vi "control - IMscram - increment buttons.vi"() -> ()   [LabVIEW 2017]
uses:
  <vilib>/imath/engines/lvmath2/RunTimeEngine/Managers/WorkSpace/UID Generator.vi
  Documents/LabVIEW Data/MathScriptVIs/MCStatic_38597427832_24a4e2d6858359c1fa390f3b06d361fe.vi
  <instcachedir>/0/MCStatic_38597427832_24a4e2d6858359c1fa390f3b06d361fe_53CC8FBD344742A8B22F0400F764026F.lvgen/MCStatic_38597427832_24a4e2d6858359c1fa390f3b06d361fe_53CC8FBD344742A8B22F0400F764026F_000.vi
  <vilib>/imath/engines/lvmath2/RunTimeEngine/RunTimeType/NIMS_RunTimeType_From StrictType (excl LVString).vi
  <instcachedir>/0/NIMS_RunTimeType_From StrictType (excl LVString)_1019F277F0A747EDBCA0F6C52CA54500.lvgen/NIMS_RunTimeType_From StrictType (excl LVString)_1019F277F0A747EDBCA0F6C52CA54500_000.vi
  <vilib>/imath/engines/lvmath2/RunTimeEngine/RunTimeType/NIMS_RunTimeType_Set Source Original Bool.vi
  <vilib>/imath/engines/lvmath2/RunTimeEngine/LocalVariableDefStatement/MC_LocalVariableDefStatement_Display.vi
  <vilib>/imath/engines/lvmath2/RunTimeEngine/Managers/SymbolTable/Clear UID.vi
  <vilib>/imath/engines/lvmath2/RunTimeEngine/NodeEndStatement/NIMS_NodeEndStatement_Output.vi
  <instcachedir>/0/NIMS_NodeEndStatement_Output_53EC0D466D134D7ABD903AC30B43404B.lvgen/NIMS_NodeEndStatement_Output_53EC0D466D134D7ABD903AC30B43404B_001.vi
  <instcachedir>/0/NIMS_NodeEndStatement_Output_53EC0D466D134D7ABD903AC30B43404B.lvgen/NIMS_NodeEndStatement_Output_53EC0D466D134D7ABD903AC30B43404B_010.vi
  <instcachedir>/0/NIMS_NodeEndStatement_Output_53EC0D466D134D7ABD903AC30B43404B.lvgen/NIMS_NodeEndStatement_Output_53EC0D466D134D7ABD903AC30B43404B_002.vi
  <vilib>/imath/engines/lvmath2/RunTimeEngine/ErrorHandling/NIMS_Finalize Error.vi
  Documents/LabVIEW Data/MathScriptVIs/MCStatic_38597427832_80100019c1ecfa069c897e41bc996adc.vi
  <instcachedir>/0/MCStatic_38597427832_80100019c1ecfa069c897e41bc996adc_8B88C90F0EB544718CCB48C9924978D1.lvgen/MCStatic_38597427832_80100019c1ecfa069c897e41bc996adc_8B88C90F0EB544718CCB48C9924978D1_001.vi
  Documents/LabVIEW Data/read2.m
  Documents/LabVIEW Data/reactor_power.m
  Documents/LabVIEW Data/long_term_power.m
  Documents/LabVIEW Data/power_function.m
  <vilib>/imath/engines/lvmath2/RunTimeEngine/Managers/SymbolTable/NIMS_WorkSpace.lvlib
panel:
  in  "Select Operation Mode":i32
  in  "Power Output On":bool
  out "Power":dbl
  out "BT-11":sgl
  out "ST-13":sgl
  out "Max k Value":dbl
  out "k value":dbl
  out "Reactivity":dbl
  in  "Fine":bool
  out "Waveform Chart":dbl(graph)
  out "Increasing?":bool
  in  "Decrease":bool
  out "Decreasing?":bool
  in  "Increase":bool
  out "Time (s)":dbl caption="Elapsed Time (s)"
  out "Iteration":i32
  out "Controlled rods out":dbl
  out "Go Scram":bool
  out "Time Satisfied":bool
  out "on":bool
  out "reset":dbl
  in  "Scram":bool
  out "Delta Satisfied":bool
  out "IM delta":dbl
  out "IM Scram Mechanism":dbl[][](array[numeric])
  out "Control Rods Positioning":dbl[][](array[numeric])
  out "Rods out":dbl format="%#_9g"
  out "Max rods out":dbl format="%#_9g"
  in  "Stop":bool
  # "MAIN WINDOW"
  # "Actual Values"
  # "Maximum Values"
  # "0 = Resistance Feedback\n2 = Shutdown"
  # "Double tap & hold"
  # "Averages"
  # "Hard1"
  # "Med1"
  # "Soft1"
  # "Hard2"
  # "Med2"
  # "Soft2"
  # "Hard3"
  # "Med3"
  # "Soft3"
  # "Initiator"
  # "Mover"
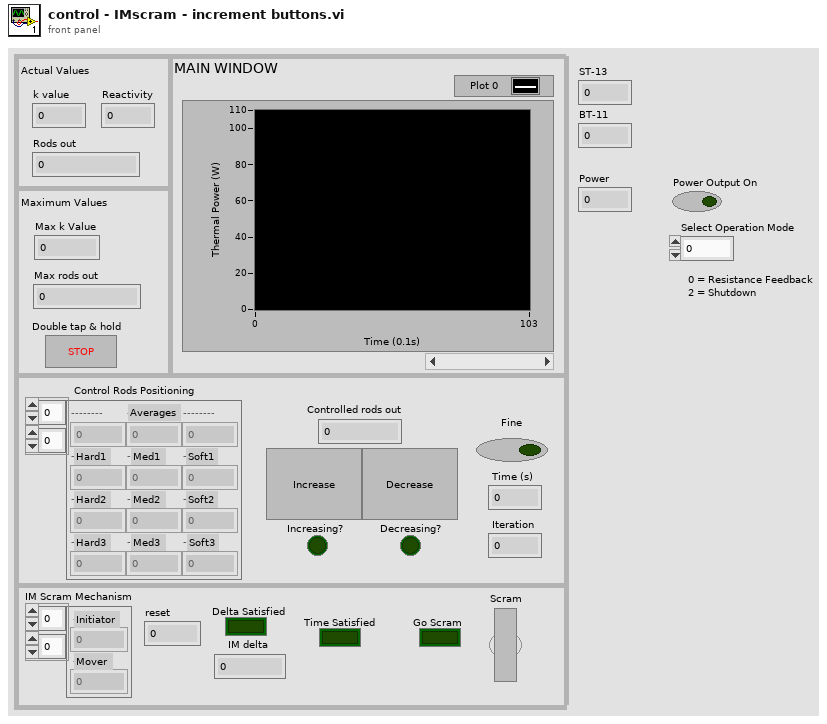
[diagram p1: front panel]
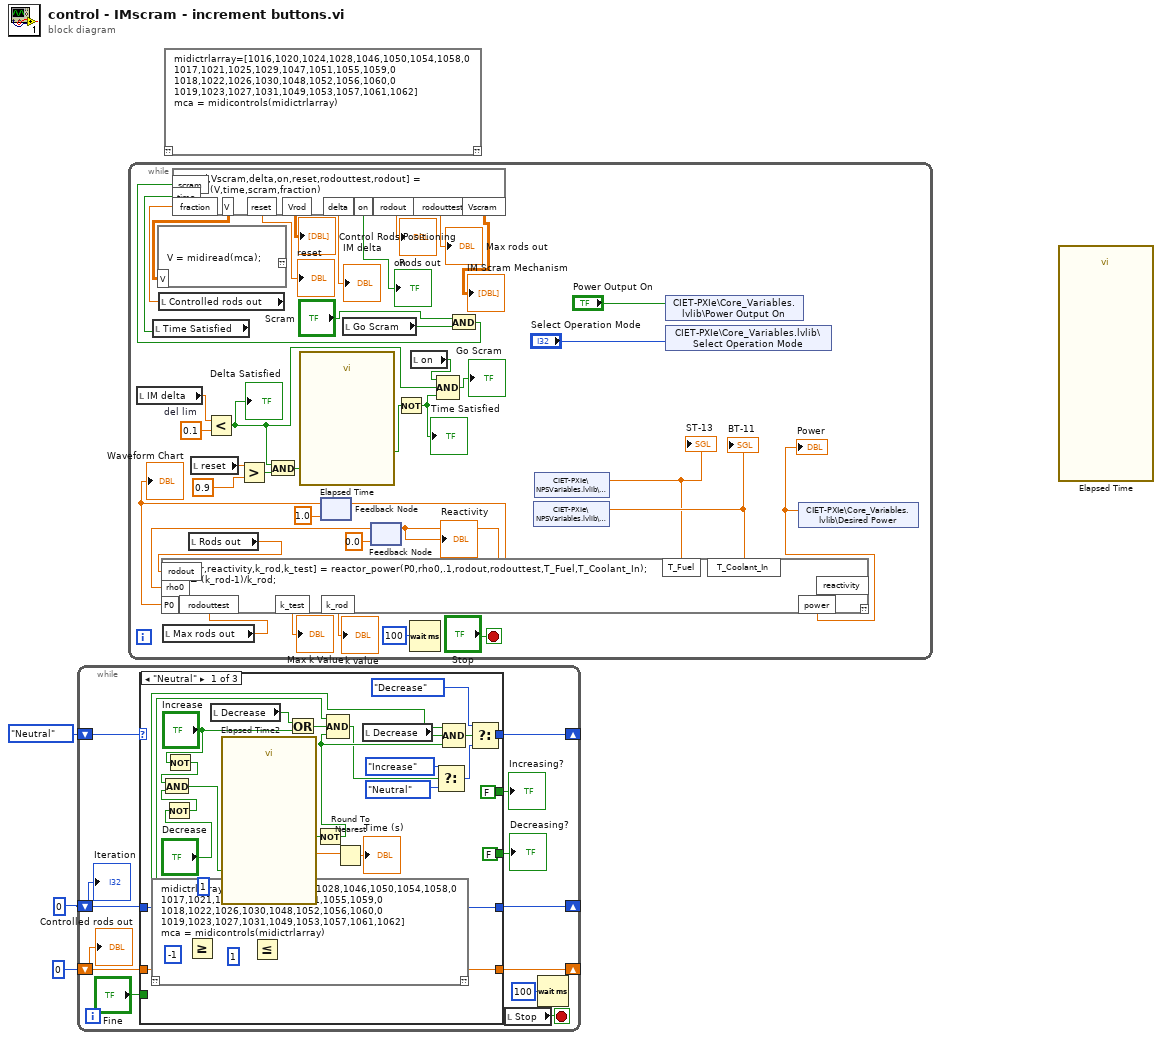
[diagram p0: block diagram]
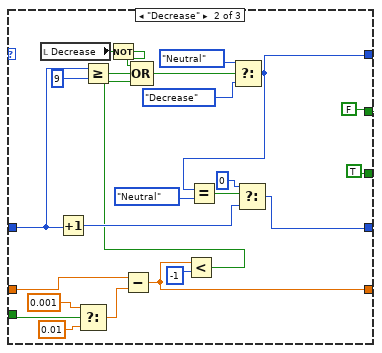
[diagram p2: hidden frame]
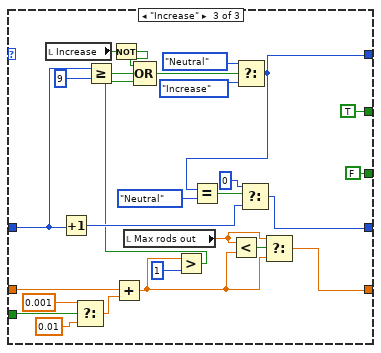
[diagram p3: hidden frame]
diagram:
  n1 = while {
    shift-right: [w12] -> _
    shift-left: enum16{"Increase", "Neutral", "Decrease"}."Neutral" -> [w13]
    shift-right: [w10] -> _
    shift-left: 0 -> [w11]
    shift-right: [w5] -> _
    shift-left: 0 -> [w8]
    stop <- w9 stop-if-true
    n2 = case shown="\"Neutral\"" w13 {
      tunnel: [w33 w49 w86] -> w12
      tunnel: w11 -> [w39 w51 w92]
      tunnel: [w39 w50 w84] -> w10
      tunnel: w8 -> [w15 w47 w69]
      tunnel: [w15 w48 w72] -> w5
      tunnel: [FALSE FALSE TRUE] -> w7
      tunnel: [FALSE TRUE FALSE] -> w6
      tunnel: "Fine" -> [_ w44 w68]
      frame "Neutral" {
        n3 = Not(x="Decrease") -> (.not. x?=w32:bool)
        n4 = Not(x="Increase") -> (.not. x?=w34:bool)
        n5 = And(x=w34, y=w32) -> (x .and. y?=w30:bool)
        n6 = Greater Or Equal?(x=w15, y=-1) -> (x >= y?=w17:bool)
        n7 = local read "Decrease"() -> (w24:bool)
        n8 = call "Elapsed Time2"("Time Target (s)"=1, "Reset"=w30) -> ("Elapsed Time (s)"=w38:dbl, "Time has Elapsed"=w40:bool)  [unwired: 10 in, 6 out]
        n9 = Less Or Equal?(x=w15, y=1) -> (x <= y?=w21:bool)
        n10 = Or(x=w24, y="Increase") -> (x .or. y?=w23:bool)
        n11 = Not(x=w40) -> (.not. x?=w20:bool)
        n12 = Compound Arithmetic op=AND(w21, w23, w20) -> (w18:bool)
        n13 = Round To Nearest(number=w38) -> (nearest integer value=→"Time (s)":dbl)
        n14 = local read "Decrease"() -> (w19:bool)
        n15 = Select(t=enum16{"Increase", "Neutral", "Decrease"}."Increase", s=w18, f=enum16{"Increase", "Neutral", "Decrease"}."Neutral") -> (s? t:f=w26:enum16{"Increase", "Neutral", "Decrease"})
        n16 = Compound Arithmetic op=AND(w17, w19, w20) -> (w22:bool)
        n17 = Select(t=enum16{"Increase", "Neutral", "Decrease"}."Decrease", s=w22, f=w26) -> (s? t:f=w33:enum16{"Increase", "Neutral", "Decrease"})
      }
      frame "Decrease" {
        n18 = local read "Decrease"() -> (w60:bool)
        n19 = Increment(x=w51) -> (x+1=w63:i32)
        n20 = Select(t=0.001, s=w44, f=0.01) -> (s? t:f=w43:dbl)
        n21 = Greater Or Equal?(x=w51, y=9) -> (x >= y?=w58:bool)
        n22 = Not(x=w60) -> (.not. x?=w59:bool)
        n23 = Subtract(x=w47, y=w43) -> (x-y=w48:dbl)
        n24 = Less?(x=w48, y=-1) -> (x < y?=w55:bool)
        n25 = Compound Arithmetic op=OR(w59, w58, w55) -> (w57:bool)
        n26 = Select(t=enum16{"Increase", "Neutral", "Decrease"}."Neutral", s=w57, f=enum16{"Increase", "Neutral", "Decrease"}."Decrease") -> (s? t:f=w49:enum16{"Increase", "Neutral", "Decrease"})
        n27 = Equal?(x=w49, y=enum16{"Increase", "Neutral", "Decrease"}."Neutral") -> (x = y?=w62:bool)
        n28 = Select(t=0, s=w62, f=w63) -> (s? t:f=w50:i32)
      }
      frame "Increase" {
        n29 = local read "Increase"() -> (w83:bool)
        n30 = Increment(x=w92) -> (x+1=w89:i32)
        n31 = Select(t=0.001, s=w68, f=0.01) -> (s? t:f=w67:dbl)
        n32 = Greater Or Equal?(x=w92, y=9) -> (x >= y?=w81:bool)
        n33 = Not(x=w83) -> (.not. x?=w82:bool)
        n34 = Add(x=w69, y=w67) -> (x+y=w73:dbl)
        n35 = local read "Max rods out"() -> (w74:dbl)
        n36 = Greater?(x=w73, y=1) -> (0:w78:bool)
        n37 = Compound Arithmetic op=OR(w82, w81, w78) -> (w80:bool)
        n38 = Less?(x=w74, y=w73) -> (x < y?=w75:bool)
        n39 = Select(t=enum16{"Increase", "Neutral", "Decrease"}."Neutral", s=w80, f=enum16{"Increase", "Neutral", "Decrease"}."Increase") -> (s? t:f=w86:enum16{"Increase", "Neutral", "Decrease"})
        n40 = Equal?(x=w86, y=enum16{"Increase", "Neutral", "Decrease"}."Neutral") -> (x = y?=w88:bool)
        n41 = Select(t=0, s=w88, f=w89) -> (s? t:f=w84:i32)
        n42 = Select(t=w74, s=w75, f=w73) -> (s? t:f=w72:dbl)
      }
    }
    "Increasing?" <- w7
    "Decreasing?" <- w6
    n43 = local read "Stop"() -> (w9:bool)
    n44 = Wait (ms)(milliseconds to wait=u32 100) -> ()  [unwired: 1 out]
    "Iteration" <- w11
    "Controlled rods out" <- w8
  }
  n45 = while {
    stop <- "Stop" stop-if-true
    w130 = 0.1  # del lim
    n46 = local read "IM delta"() -> (w131:dbl)
    n47 = local read "Time Satisfied"() -> (w116:bool)
    n48 = script code="V = midiread(mca);"() -> ("V"=w117:dbl[][])  [unwired: 1 in, 1 out]
    n49 = local read "Controlled rods out"() -> (w103:dbl)
    n50 = local read "Max rods out"() -> (w100:dbl)
    n51 = local read "Rods out"() -> (w104:dbl)
    n52 = local read "reset"() -> (w126:dbl)
    n53 = Less?(x=w131, y=w130) -> (x < y?=w110:bool)
    "Delta Satisfied" <- w110
    n54 = Greater?(x=w126, y=0.9) -> (0:w125:bool)
    n55 = And(x=w110, y=w125) -> (x .and. y?=w127:bool)
    n56 = call "Elapsed Time"("Reset"=w127) -> ("Time has Elapsed"=w128:bool)  [unwired: 11 in, 7 out]
    n57 = feedback #1(1.0 ("power")) -> (w105:dbl)
    "Waveform Chart" <- w105
    n58 = local read "Go Scram"() -> (w123:bool)
    n59 = feedback #2(0.0 ("reactivity")) -> (w108:dbl)
    n60 = Not(x=w128) -> (.not. x?=w115:bool)
    "Time Satisfied" <- w115
    n61 = Wait (ms)(milliseconds to wait=100) -> ()  [unwired: 1 out]
    n62 = local read "on"() -> (w112:bool)
    n63 = Compound Arithmetic op=AND(w112, w110, w115) -> (→"Go Scram":bool)
    n64 = And(x="Scram", y=w123) -> (x .and. y?=w109:bool)
    n65 = mathscript code="[Vrod,Vscram,delta,on,reset,rodouttest,rodout] = read2(V,time,scram,fraction)"("V"=w117, "scram"=w109, "time"=w116, "fraction"=w103) -> ("rodout"=→"Rods out":dbl, "rodouttest"=→"Max rods out":dbl, "Vrod"=→"Control Rods Positioning":dbl[][], "Vscram"=→"IM Scram Mechanism":dbl[][], "delta"=→"IM delta":dbl, "on"=→"on":bool, "reset"=→"reset":dbl)  [unwired: 1 in, 1 out]
    n66 = shared-variable "CIET-PXIe\\NPSVariables.lvlib\\BT-11"() -> (w98:sgl)  [unwired: 1 in, 1 out]
    "BT-11" <- w98
    n67 = shared-variable "CIET-PXIe\\NPSVariables.lvlib\\ST-13"() -> (w97:sgl)  [unwired: 1 in, 1 out]
    "ST-13" <- w97
    n68 = mathscript code="[power,reactivity,k_rod,k_test] = reactor_power(P0,rho0,.1,rodout,rodouttest,T_Fuel,T_Coolant_In);\nrho = (k_rod-1)/k_rod;"("P0"=w105, "rho0"=w108, "rodout"=w104, "rodouttest"=w100, "T_Fuel"=w97, "T_Coolant_In"=w98) -> ("power"=w96:dbl, "reactivity"=w102:dbl, "k_rod"=→"k value":dbl, "k_test"=→"Max k Value":dbl)  [unwired: 1 in, 1 out]
    "Reactivity" <- w102
    "Power" <- w96
    n69 = feedback-in #1(w96) -> ()
    n70 = feedback-in #2(w102) -> ()
    n71 = shared-variable "CIET-PXIe\\Core_Variables.lvlib\\Power Output On"("Power Output On") -> ()  [unwired: 1 in, 1 out]
    n72 = shared-variable "CIET-PXIe\\Core_Variables.lvlib\\Select Operation Mode"("Select Operation Mode") -> ()  [unwired: 1 in, 1 out]
    n73 = shared-variable "CIET-PXIe\\Core_Variables.lvlib\\Desired Power"(w96) -> ()  [unwired: 1 in, 1 out]
  }
  n74 = script code="midictrlarray=[1016,1020,1024,1028,1046,1050,1054,1058,0\n1017,1021,1025,1029,1047,1051,1055,1059,0\n1018,1022,1026,1030,1048,1052,1056,1060,0\n1019,1023,1027,1031,1049,1053,1057,1061,1062]\nmca = midicontrols(midictrlarray)"() -> ()  [unwired: 1 in, 1 out]
  n75 = script code="midictrlarray=[1016,1020,1024,1028,1046,1050,1054,1058,0\n1017,1021,1025,1029,1047,1051,1055,1059,0\n1018,1022,1026,1030,1048,1052,1056,1060,0\n1019,1023,1027,1031,1049,1053,1057,1061,1062]\nmca = midicontrols(midictrlarray)"() -> ()  [unwired: 1 in, 1 out]
  n76 = call "Elapsed Time"() -> ()  [unwired: 12 in, 8 out]
